vi "testRio.vi"() -> ()   [LabVIEW 2015]
uses:
  Library/IF2_Reader/IF2_Reader.lvlib
panel:
  in  "Developer pass":string
  out "TagArray":string[](array[string])
  out "TagData out":cluster{"TagCode":string, "FirstSeemUs":u64}[](array[cluster])
  out "Report":string
  in  "stop":bool
  out "parar":bool
  in  "OK Button":bool
  out "OK Button 2":bool
  out "connection ID":refnum<k5>
  in  "IP RFID":string="172.23.3.203"
  in  "Puerto RFID":u16=2189
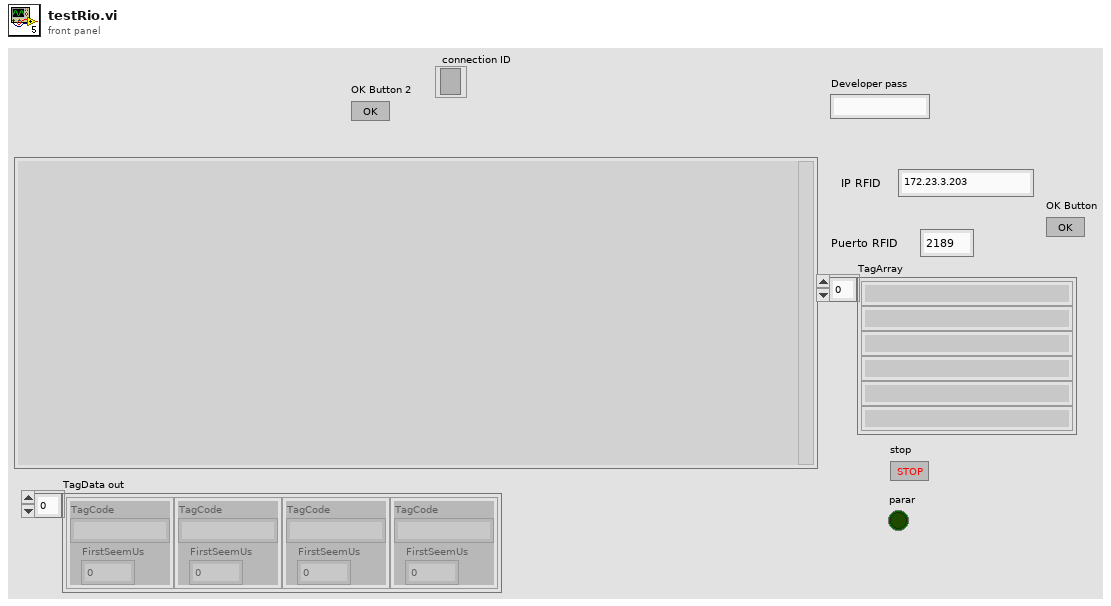
[diagram p1: front panel]
types:
  T1 = cluster{"IP":string, "Port":u16, "ReaderConfigFile":path, "ROspecConfigFile":path}
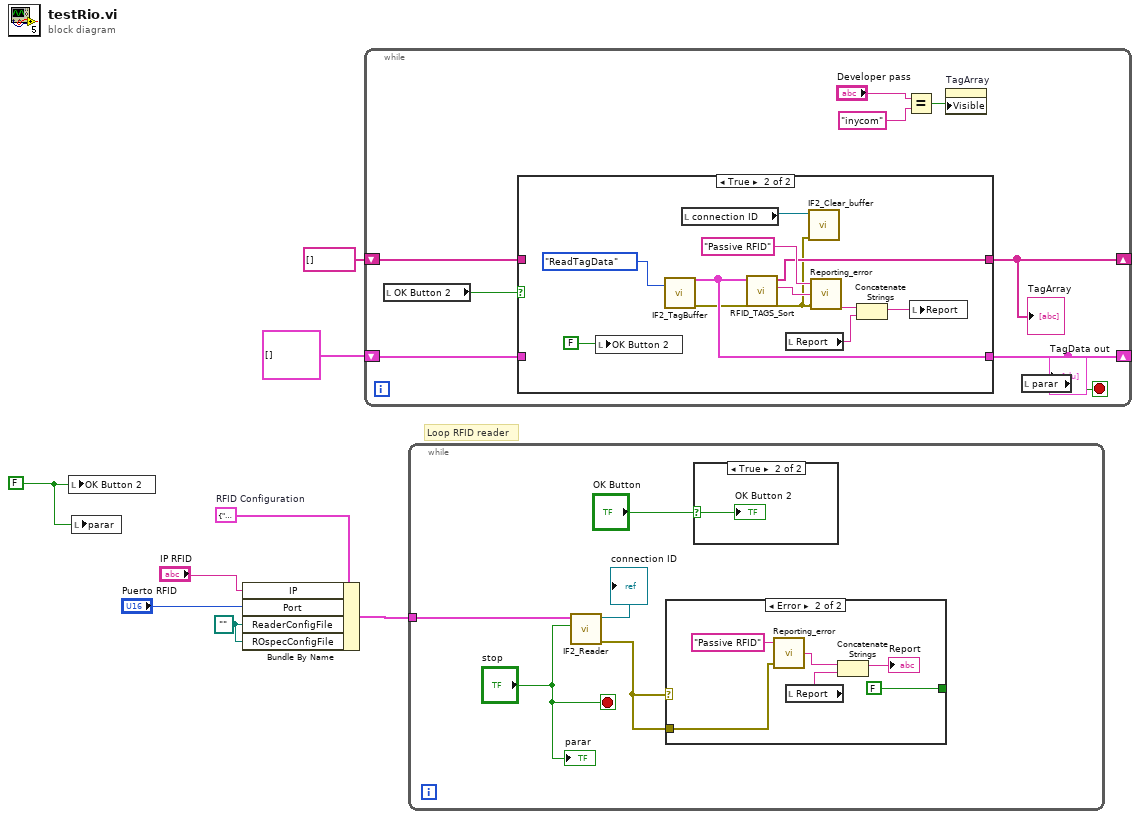
[diagram p0: block diagram]
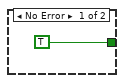
[diagram p4: hidden frame]
diagram:
  w3 = FALSE ("Boolean")
  w8 = T1 {"IP"="169.254.1.1", "Port"=5084, "ReaderConfigFile"=path "", "ROspecConfigFile"=path ""}  # RFID Configuration
  w6 = path "" ("ReaderConfigFile")
  # "Loop RFID reader"
  n1 = local write "OK Button 2"(w3) -> ()
  n2 = local write "parar"(w3) -> ()
  n3 = Bundle By Name(cluster=w8, "IP"="IP RFID", "Port"="Puerto RFID", "ReaderConfigFile"=w6, "ROspecConfigFile"=w6) -> (w7:T1)
  n4 = while {
    shift-right: [w15] -> _
    shift-left: string[] [] ("TagArray") -> [w14]
    shift-right: [w13] -> _
    shift-left: cluster{"TagCode":string, "FirstSeemUs":u64}[] [] ("TagData out") -> [w12]
    stop <- w17 stop-if-true
    n5 = local read "OK Button 2"() -> (w16:bool)
    n6 = case shown="True" w16 {
      tunnel: [w19 w24] -> w15
      tunnel: [w18 w23] -> w13
      tunnel: w14 -> [w19 _]
      tunnel: w12 -> [w18 _]
      frame False {
      }
      frame True {
        n7 = local write "OK Button 2"(FALSE ("Boolean")) -> ()
        n8 = call "IF2_TagBuffer.vi"("Action"=enum16{"Init", "WriteTagData", "ReadTagData"}."ReadTagData") -> ("error out"=w21:errorcluster, "TagData out"=w23:cluster{"TagCode":string, "FirstSeemUs":u64}[])  [unwired: 9 in]
        n9 = local read "connection ID"() -> (w20:refnum<k5>)
        n10 = call "RFID_TAGS_Sort.vi"("TagData in"=w23) -> ("TagString"=w25:string, "TagArray"=w24:string[])  [unwired: 9 in]
        n11 = local read "Report"() -> (w26:string)
        n12 = call "IF2_Clear_buffer.vi"("error in (no error)"=w21, "TCP Network Connection in"=w20) -> ()  [unwired: 8 in, 2 out]
        n13 = call "Reporting_error.vi"("error out 2"=w21, "Concept explanation"=w25, "Concept"="Passive RFID") -> ("Reporting"=w29:string)
        n14 = Concatenate Strings(w29, w26) -> (w27:string)
        n15 = local write "Report"(w27) -> ()
      }
    }
    "TagArray" <- w15
    "TagData out" <- w13
    n16 = Equal?(x="Developer pass", y="inycom") -> (x = y?=w11:bool)
    n17 = property on="TagArray" class="Arr (strict)"("Visible"=w11) -> ()  [unwired: 2 in, 2 out]
    n18 = local read "parar"() -> (w17:bool)
  }
  n19 = while {
    tunnel: w7 -> [w34]
    stop <- "stop" stop-if-true
    n20 = call "IF2_Reader.vi"("Stop"="stop", "RFID Configuration"=w34) -> ("error out"=w35:errorcluster, "connection ID"=→"connection ID":refnum<k5>)  [unwired: 8 in]
    n21 = case shown="Error" w35 {
      tunnel: w35 -> [_ w39]
      tunnel: [TRUE ("RFIDStatus") FALSE ("RFIDStatus")] -> _
      frame No Error {
      }
      frame Error {
        n22 = call "Reporting_error.vi"("error out 2"=w39, "Concept"="Passive RFID") -> ("Reporting"=w40:string)  [unwired: 1 in]
        n23 = local read "Report"() -> (w41:string)
        n24 = Concatenate Strings(w40, w41) -> (→"Report":string)
      }
    }
    n25 = case shown="True" "OK Button" {
      selector: "OK Button" -> [_ w36]
      frame False {
      }
      frame True {
        "OK Button 2" <- w36
      }
    }
    "parar" <- "stop"
  }
